vi "Adjust Dashboard Window.vi"(6 "Sizing Refnums":T1, 9 "Size Constraints":cluster{"min tab width":i32, "w/h":dbl}, 10 "VI":refnum<vi>, 11 "Notifier in":refnum<notifier>) -> ()   [LabVIEW 2014]
uses:
  <vilib>/Utility/miscctls.llb/LVRectTypeDef.ctl
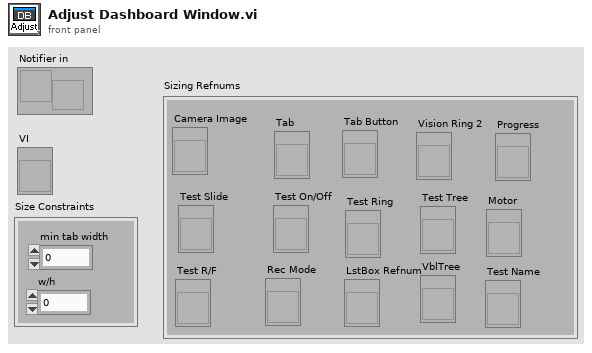
[diagram p1: front panel]
types:
  T1 = cluster{"Camera Image":refnum<vi>, "Tab":refnum<vi>, "Tab Button":refnum<vi>, "Vision Ring 2":refnum<vi>, "Rec Mode":refnum<vi>, "Test Slide":refnum<vi>, "Test On/Off":refnum<vi>, "Test Ring":refnum<vi>, "Test R/F":refnum<vi>, "Test Name":refnum<vi>, "Motor":refnum<vi>, "Progress":refnum<vi>, "LstBox Refnum":refnum<vi>, "Test Tree":refnum<vi>, "VblTree":refnum<vi>}
  T2 = typedef "LVRectTypeDef.ctl" = cluster{"Left":i16, "Top":i16, "Right":i16, "Bottom":i16}
  T3 = typedef "LVPointTypeDef.ctl" = cluster{"Horizontal":i16, "Vertical":i16}
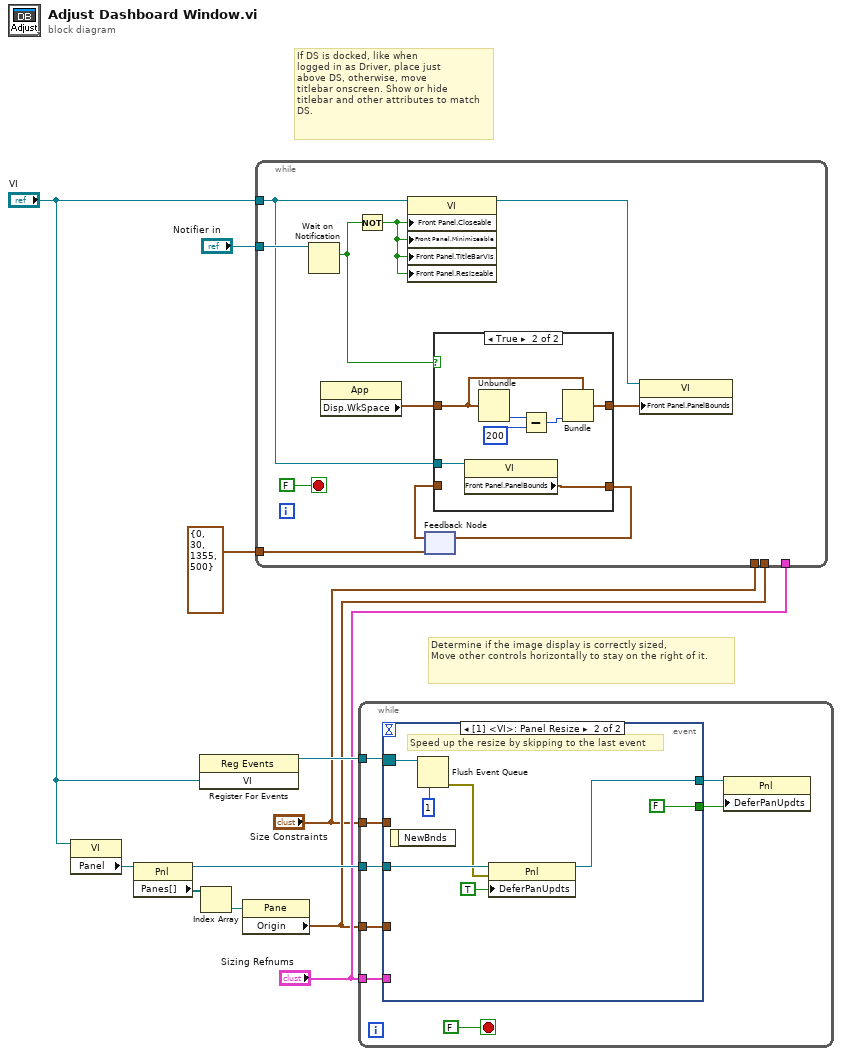
[diagram p0: block diagram]
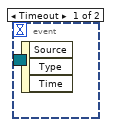
[diagram p2: hidden frame]
diagram:
  # "Determine if the image display is correctly sized,\nMove other controls horizontally to stay on the right of it."
  # "If DS is docked, like when\nlogged in as Driver, place just\nabove DS, otherwise, move\ntitlebar onscreen. Show or hide\ntitlebar and other attributes to match\nDS."
  n1 = property class="VI"(reference="VI") -> ("Panel"=w8:refnum<vi>)  [unwired: 1 in, 2 out]
  n2 = property class="Pnl"(reference=w8) -> (reference out=w5:refnum<vi>, "Panes[]"=w7:refnum<vi>[])  [unwired: 1 in, 1 out]
  n3 = register-events("VI") -> (reference out=w10:refnum<event-registration>)  [unwired: 2 in, 1 out]
  n4 = Index Array(array=w7) -> (element=w6:refnum<vi>)  [unwired: 1 in]
  n5 = property class="Pane"(reference=w6) -> ("Origin"=w3:T3)  [unwired: 1 in, 2 out]
  n6 = while {
    tunnel: "Notifier in" -> [w21]
    tunnel: "VI" -> [w16]
    tunnel: "Sizing Refnums" -> [_]
    tunnel: w3 -> [_]
    tunnel: "Size Constraints" -> [_]
    tunnel: T2 {"Left"=0, "Top"=30, "Right"=1355, "Bottom"=500} ("Front Panel.PanelBounds") -> [w13]
    stop <- FALSE stop-if-true
    n7 = Wait on Notification(notifier=w21) -> (notification=w17:bool)  [unwired: 3 in, 3 out]
    n8 = property class="App"() -> ("Disp.WkSpace"=w20:T2)  [unwired: 2 in, 2 out]
    n9 = Not(x=w17) -> (.not. x?=w12:bool)
    n10 = property class="VI"(reference=w16, "Front Panel.Closeable"=w12, "Front Panel.Minimizeable"=w12, "Front Panel.TitleBarVis"=w12, "Front Panel.Resizeable"=w12) -> (reference out=w19:refnum<vi>)  [unwired: 1 in, 1 out]
    n11 = feedback #1(w13) -> (w14:T2)
    n12 = case shown="True" w17 {
      tunnel: w20 -> [_ w26]
      tunnel: [w23 w27] -> w18
      tunnel: w16 -> [_ w25]
      tunnel: [w23 w24] -> w15
      tunnel: w14 -> [w23 _]
      frame False {
      }
      frame True {
        n13 = property class="VI"(reference=w25) -> ("Front Panel.PanelBounds"=w24:T2)  [unwired: 1 in, 2 out]
        n14 = Unbundle(w26) -> ("Bottom"=w30:i16)  [unwired: 3 out]
        n15 = Subtract(x=w30, y=200) -> (x-y=w28:i32)
        n16 = Bundle(cluster=w26, "Bottom"=w28) -> (w27:T2)  [unwired: 3 out]
      }
    }
    n17 = feedback-in #1(w15) -> ()
    n18 = property class="VI"(reference=w19, "Front Panel.PanelBounds"=w18) -> ()  [unwired: 1 in, 2 out]
  }
  n19 = while {
    tunnel: w10 -> [w37]
    tunnel: "Sizing Refnums" -> [w36]
    tunnel: "Size Constraints" -> [w35]
    tunnel: w3 -> [w34]
    tunnel: w5 -> [w33]
    stop <- FALSE stop-if-true
    n20 = event shown="[1] <VI>: Panel Resize" {
      selector: w37 -> [_ w42]
      dyn-events: _ -> [_ _]
      timeout: _ -> [_ _]
      tunnel: w36 -> [_ _]
      tunnel: w35 -> [_ _]
      tunnel: w34 -> [_ _]
      tunnel: w33 -> [_ w45]
      tunnel: [_ FALSE ("Defer Panel Updates")] -> w32
      tunnel: [_ w39] -> w31
      event Timeout {
        n21 = event-data() -> ()  [unwired: 1 in, 3 out]
      }
      event Panel Resize {
        # "Speed up the resize by skipping to the last event"
        n22 = event-data() -> ()  [unwired: 1 in, 1 out]
        n23 = Flush Event Queue(0:w42, 5:1 ("keep most recent")) -> (11:w40:errorcluster)  [unwired: 4 in, 2 out]
        n24 = property class="Pnl"(reference=w45, error in=w40, "DeferPanUpdts"=TRUE ("Defer Panel Updates")) -> (reference out=w39:refnum<vi>)  [unwired: 1 out]
      }
    }
    n25 = property class="Pnl"(reference=w31, "DeferPanUpdts"=w32) -> ()  [unwired: 1 in, 2 out]
  }
